vi "REACTOR_MODO AUTOM.vi"(7 "Secuencia":string[](array[string]), 8 "error in (no error)":errorcluster, 9 "ALICATS":T4=[["3", "NO", "M0000013", "Air", "10", "ln/mn", "0", "0"], ["4", "NO", "M0000014", "Air", "10", "ln/mn", "0", "0"], ["5", "NO", "M0000015", "Air", "10", "ln/mn", "0", "0"], ["6", "NO", "M0000016", "Air", "10", "ln/mn", "0", "0"], ["7", "NO", "M0000017", "Air", "10", "ln/mn", "0", "0"], ["8", "NO", "M0000018", "Air", "10", "ln/mn", "0", "0"]], 10 "Eurotherm":T1, 11 "Comms":T5={"Alicats"="ASRL6::INSTR", "Alic"=FALSE, "eValve"="ASRL6::INSTR", "eval"=FALSE, "Eurotherm"="ASRL6::INSTR", "euro"=FALSE, "Cell GAS"="ASRL6::INSTR", "cgas"=FALSE, "Cell H2S"="ASRL6::INSTR", "ch2s"=FALSE}) -> (0 "error out":errorcluster)   [LabVIEW 2017]
uses:
  REACTOR_DATOS.ctl
  REACTOR_COMUNICACIONES.ctl
  SERIAL ALICATS/__s_TablaAlicats.ctl
  EUROTHERM/TEG P116x2.ctl
  EUROTHERM/2xP116.ctl
  SERIAL ALICATS/__Alicat SD_ReadingCluster.ctl
  DISPLAY/Data Type.ctl
  DISPLAY/Display_Command Control.ctl
  REACTOR_MODO AUTOM.ctl
  FILE/File_Module Control.ctl
  TIMING/Timing_Module Control.ctl
  SERIAL RASP_PICO VALVE/kissia_rasPico Module.ctl
  EUROTHERM/Eurotherm_New_Module.ctl
  REACTOR_GLOBALES.vi
panel:
  out "ERRORES_T 2":i32=5 caption="Elapsed Time (s)"
  out "P116x2":T1
  out "ERRORES_T":i32=5 caption="Elapsed Time (s)"
  out "tPlato(s)":dbl=1.0
  out "ParsedReadingArray":T3[](array[typedef]) {"Total" format="%.2f"; "SetPoint" format="%.2f"; "Mass" format="%.2f"; "Volumetric" format="%.2f"; "Temperature" format="%.2f"; "Pressure" format="%.2f"}
  out "T.Wait Stability":bool
  out "Mide Alicats":bool=TRUE
  out "Mide Temps":bool=TRUE
  out "Muestreo(s)":dbl=1.0
  out "TIEMPO (m)":dbl
  out "VALVULA":bool
  out "Timestring":string
  out "Max_t(s)":dbl format="%.1f"
  out "Delta t(s)":dbl format="%.1f"
  out "Delta T(C)":dbl format="%.1f"
  out "TStable":bool
  out "Datos":T6 {"a FSET4" format="%.2g"; "a FSET3" format="%.2g"; "a FSET2" format="%.2g"; "a FSET1" format="%.2g"; "a FLUJO4" format="%.2g"; "a FLUJO2" format="%.2g"; "a FLUJO1" format="%.2g"; "a FLUJO3" format="%.2g"; "eVAL_5" format="%.2g"; "TEMP_TH" format="%.2g"; "SET_TH" format="%.2g"; "TEMP_TC" format="%.2g"; "SET_TC" format="%.2g"; "TIEMPO" format="%.2g"}
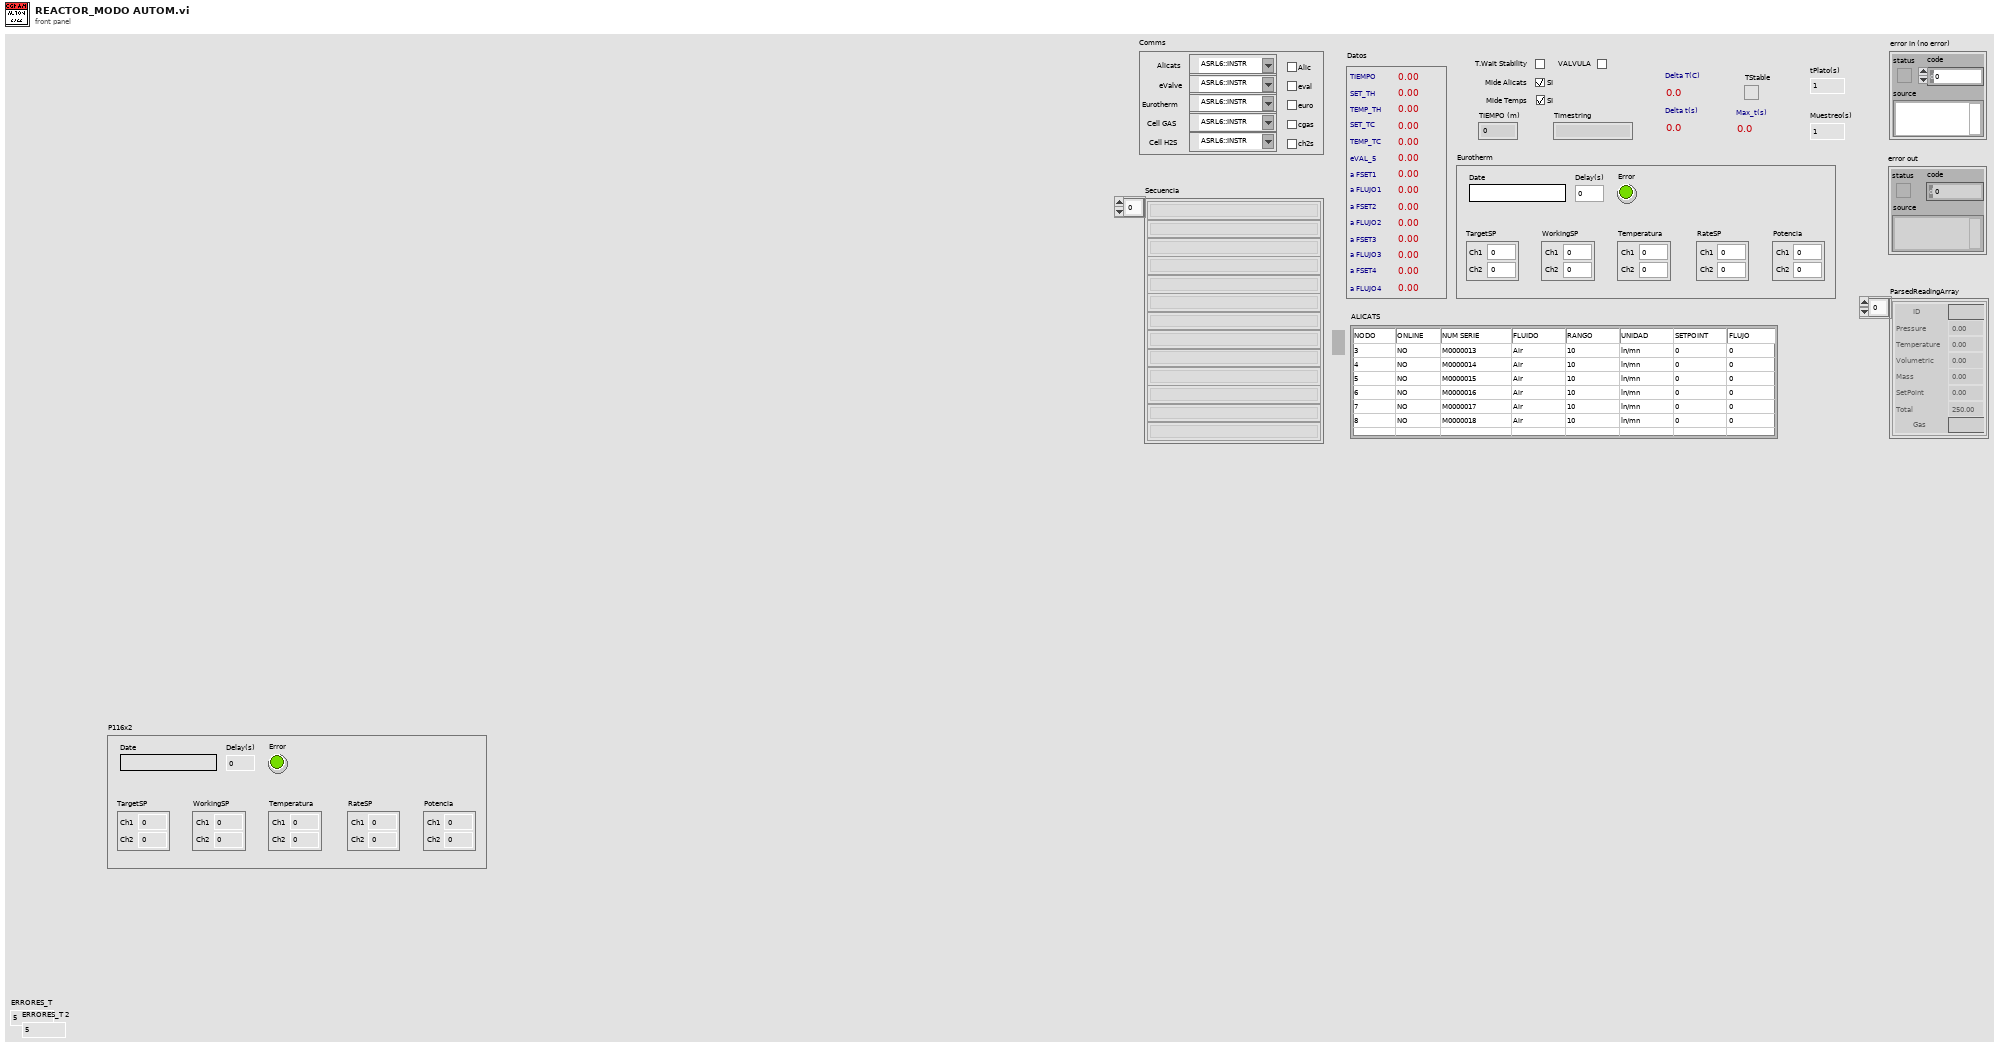
[diagram p1: front panel]
types:
  T1 = typedef "TEG P116x2.ctl" = cluster{"TargetSP":T2, "WorkingSP":T2, "Temperatura":T2, "Error":bool, "Date":string, "Delay(s)":dbl, "RateSP":T2, "Potencia":T2}
  T2 = typedef "2xP116.ctl" = cluster{"Ch1":dbl, "Ch2":dbl}
  T3 = typedef "__Alicat SD_ReadingCluster.ctl" = cluster{"ID":string, "Pressure":sgl, "Temperature":sgl, "Volumetric":sgl, "Mass":sgl, "SetPoint":sgl, "Gas":string, "Total":sgl}
  T4 = typedef "__s_TablaAlicats.ctl" = string[][]
  T5 = typedef "REACTOR_COMUNICACIONES.ctl" = cluster{"Alicats":refnum<visa-resource-name>, "Alic":bool, "eValve":refnum<visa-resource-name>, "eval":bool, "Eurotherm":refnum<visa-resource-name>, "euro":bool, "Cell GAS":refnum<visa-resource-name>, "cgas":bool, "Cell H2S":refnum<visa-resource-name>, "ch2s":bool}
  T6 = typedef "REACTOR_DATOS.ctl" = cluster{"TIEMPO":dbl, "SET_TH":dbl, "TEMP_TH":dbl, "SET_TC":dbl, "TEMP_TC":dbl, "eVAL_5":dbl, "a FSET1":dbl, "a FLUJO1":dbl, "a FSET2":dbl, "a FLUJO2":dbl, "a FSET3":dbl, "a FLUJO3":dbl, "a FSET4":dbl, "a FLUJO4":dbl}
  T7 = typedef "Data Type.ctl" = enum16{"Init FP", "En/Dis FP Ctls", "Update FP", "Upd Status", "Upd Seq"}
  T8 = typedef "Display_Command Control.ctl" = enum16{"Initialize", "Generate Event", "Shutdown"}
  T9 = typedef "REACTOR_MODO AUTOM.ctl" = enum16{"INICIALIZAR", "TEST COMANDO", "PARAMETROS MEDIDA", "CAMBIO ALICATS", "CAMBIO VALVULA", "CAMBIO TEMPERATURAS", "cTEMPERATURA ESTABLE?", "cLEER TIEMPO", "cLEER TEMPERATURAS", "cLEER ALICATS", "cGUARDAR DATOS", "cWAIT NEXT", "CAMBIO TIEMPOS", "tAGOTADO TIEMPO?", "tLEER TIEMPO", "tLEER TEMPERATURAS", "tLEER ALICATS", "tGUARDAR DATOS", "tWAIT NEXT", "FINALIZAR"}
  T10 = typedef "File_Module Control.ctl" = enum16{"Initialize", "Save Head", "Save Data", "Shutdown"}
  T11 = typedef "kissia_rasPico Module.ctl" = enum16{"Initialize", "Read Data", "Write Data", "Enable", "Disable", "Shutdown"}
  T12 = typedef "Timing_Module Control.ctl" = enum16{"Initialize Time", "Check Time"}
  T13 = typedef "Eurotherm_New_Module.ctl" = enum16{"Initialize", "Write SP", "Read SP+PV", "Write Rate", "Set P", "Set I", "Set D", "Shutdown"}
  T14 = typedef "__s_SPali4.ctl" = cluster{"Ch1":dbl, "Ch2":dbl, "Ch3":dbl, "Ch4":dbl, "Ch5":dbl, "Ch6":dbl}
  T15 = enum16{"Add 1", "Add 2", "Add 10", "Add 11", "Add 12", "Add 13"}[]
  T16 = cluster{"processVal":dbl, "targetSP":dbl, "workingSP":dbl, "workingOut":dbl}
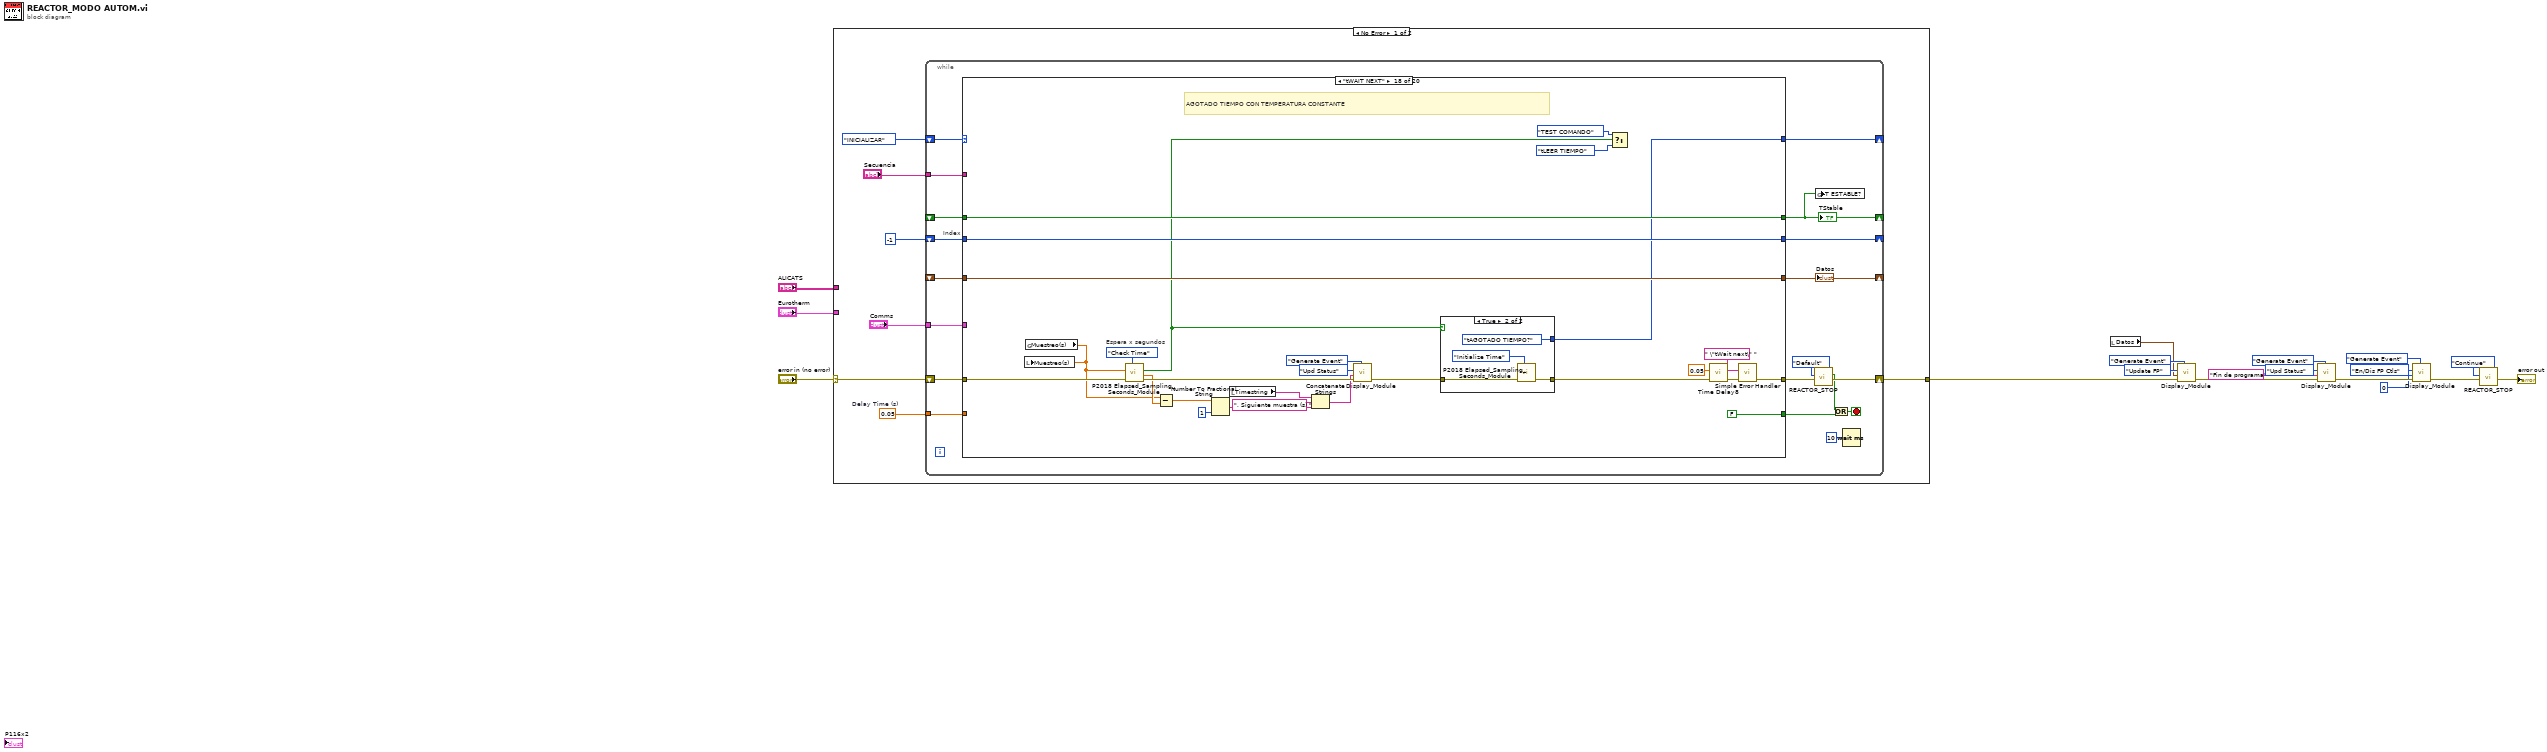
[diagram p0: block diagram]
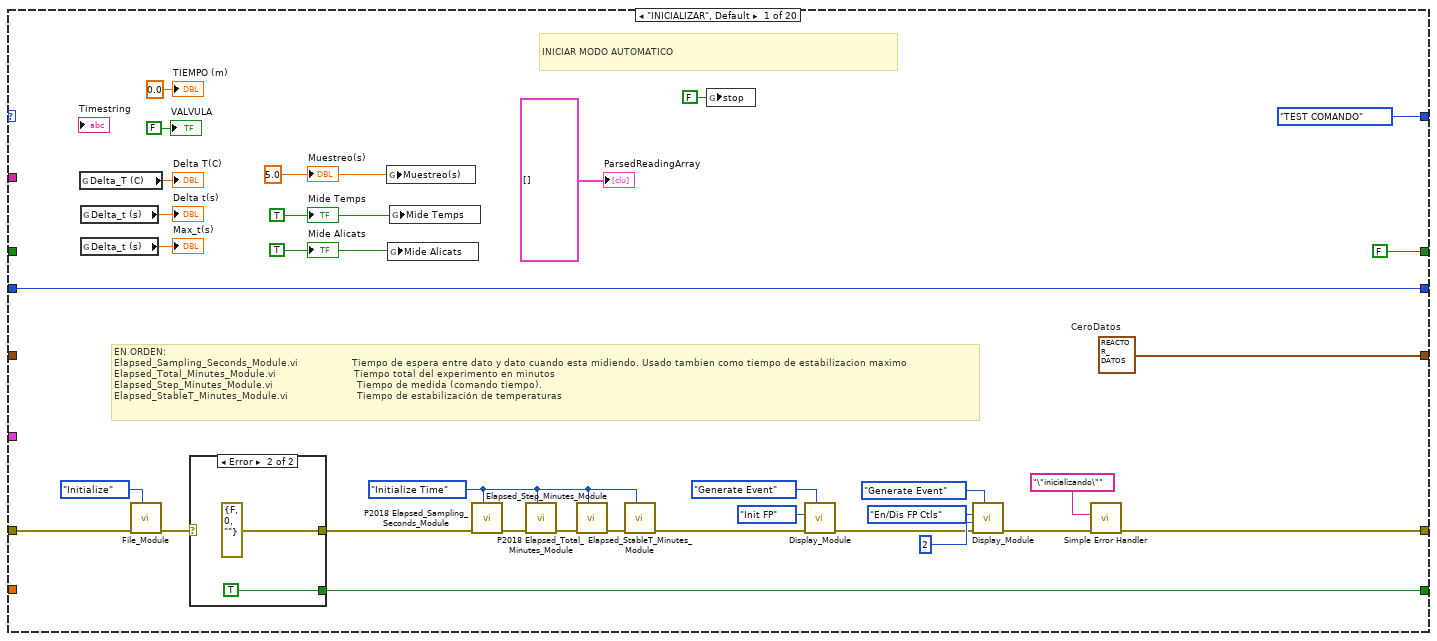
[diagram p2: hidden frame]
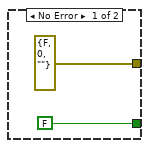
[diagram p3: hidden frame]
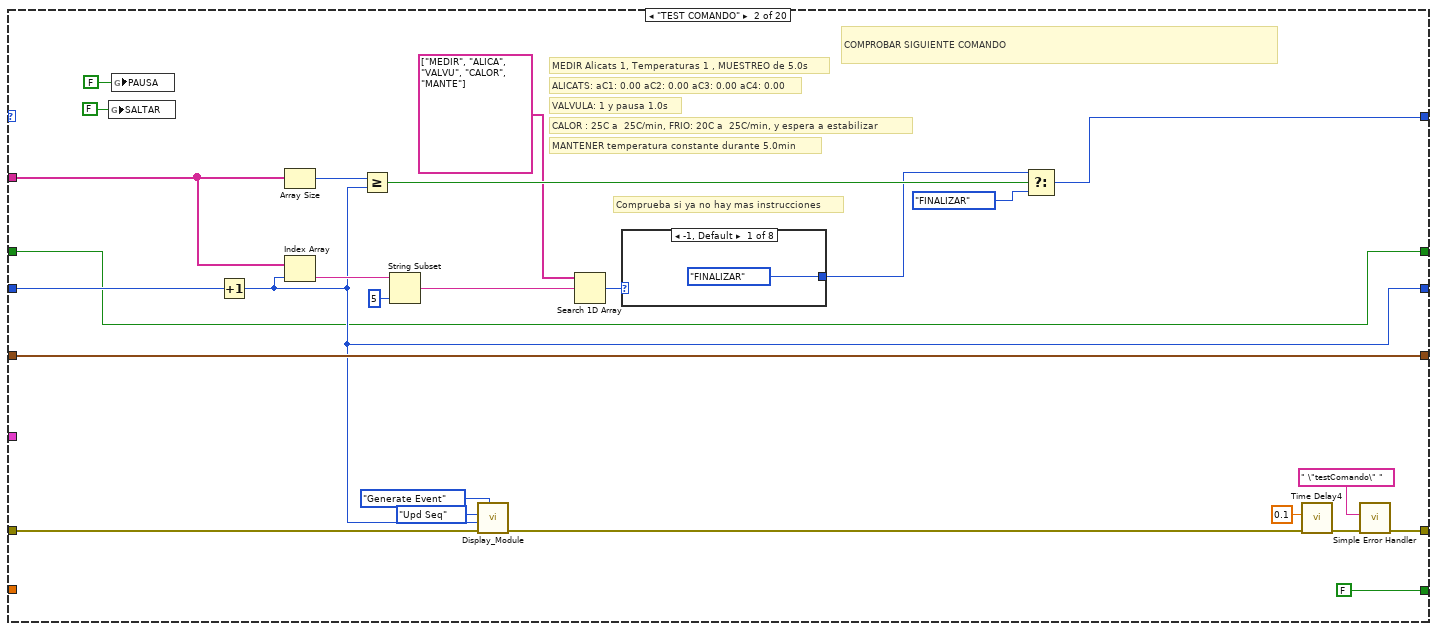
[diagram p4: hidden frame]
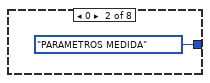
[diagram p5: hidden frame]
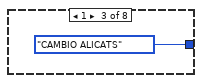
[diagram p6: hidden frame]
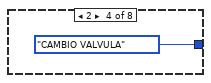
[diagram p7: hidden frame]
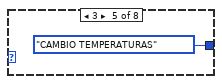
[diagram p8: hidden frame]
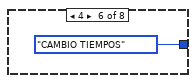
[diagram p9: hidden frame]
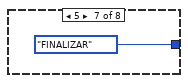
[diagram p10: hidden frame]
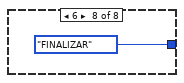
[diagram p11: hidden frame]
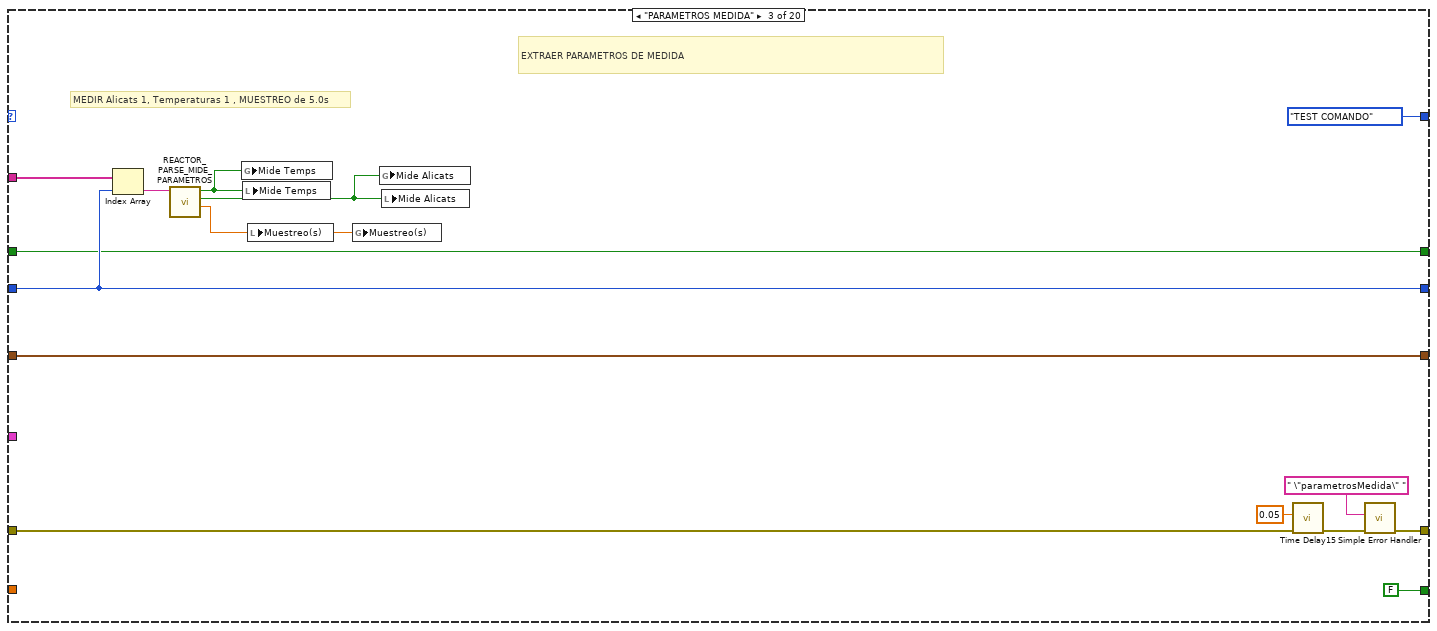
[diagram p12: hidden frame]
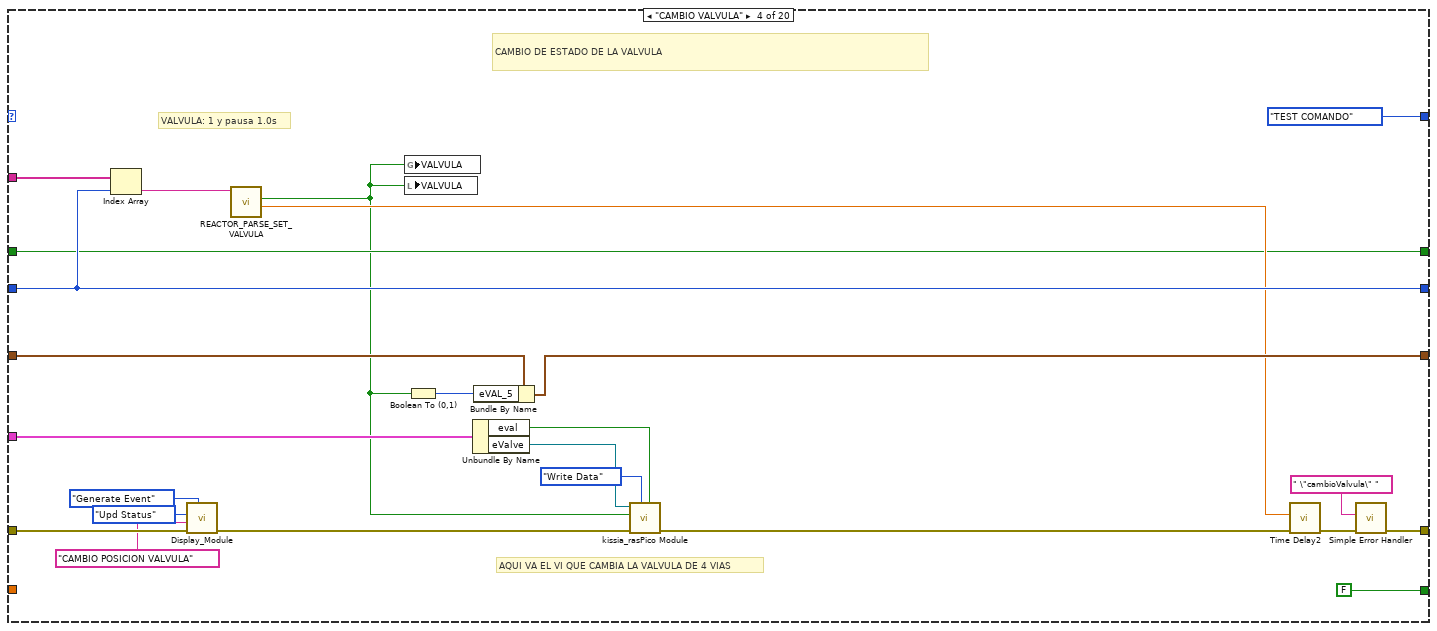
[diagram p13: hidden frame]
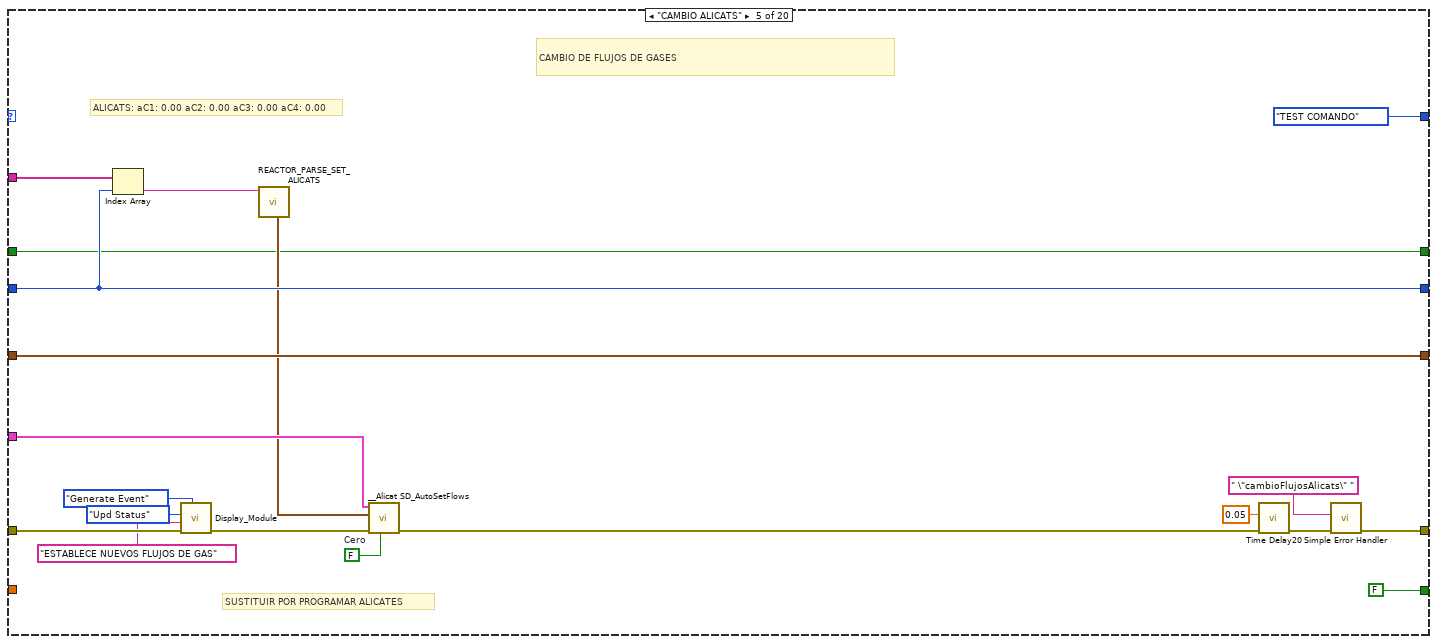
[diagram p14: hidden frame]
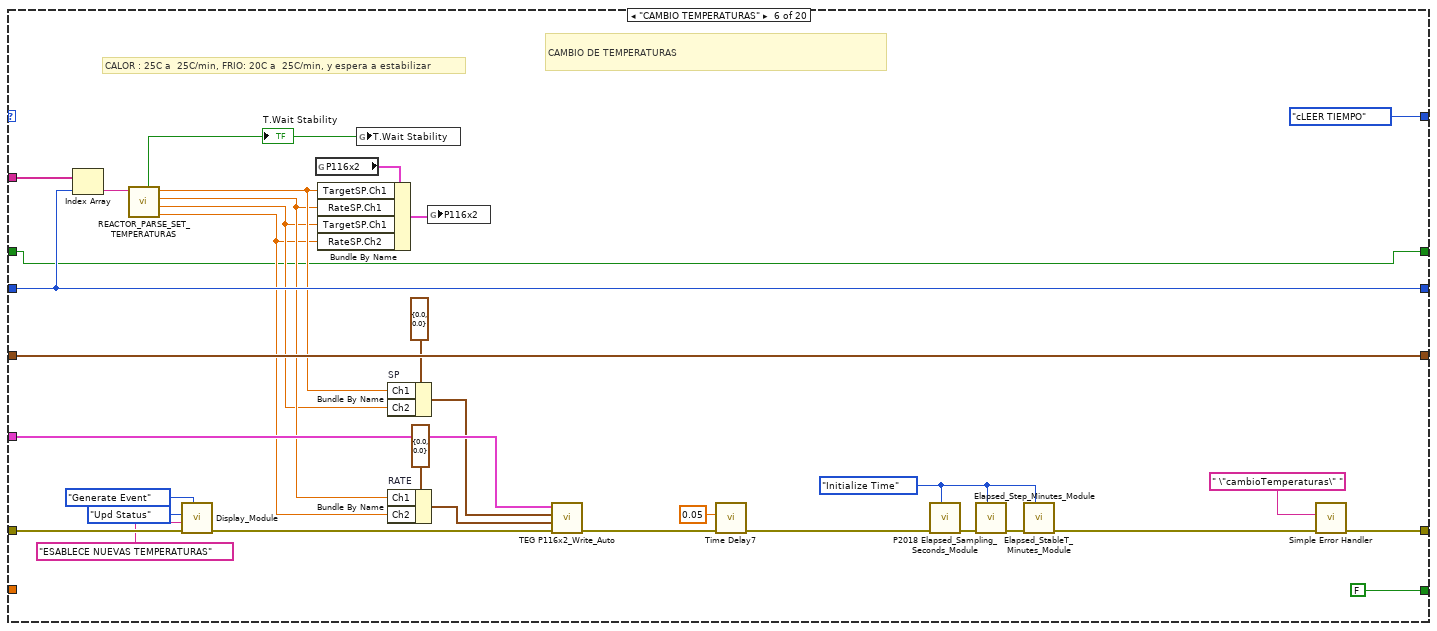
[diagram p15: hidden frame]
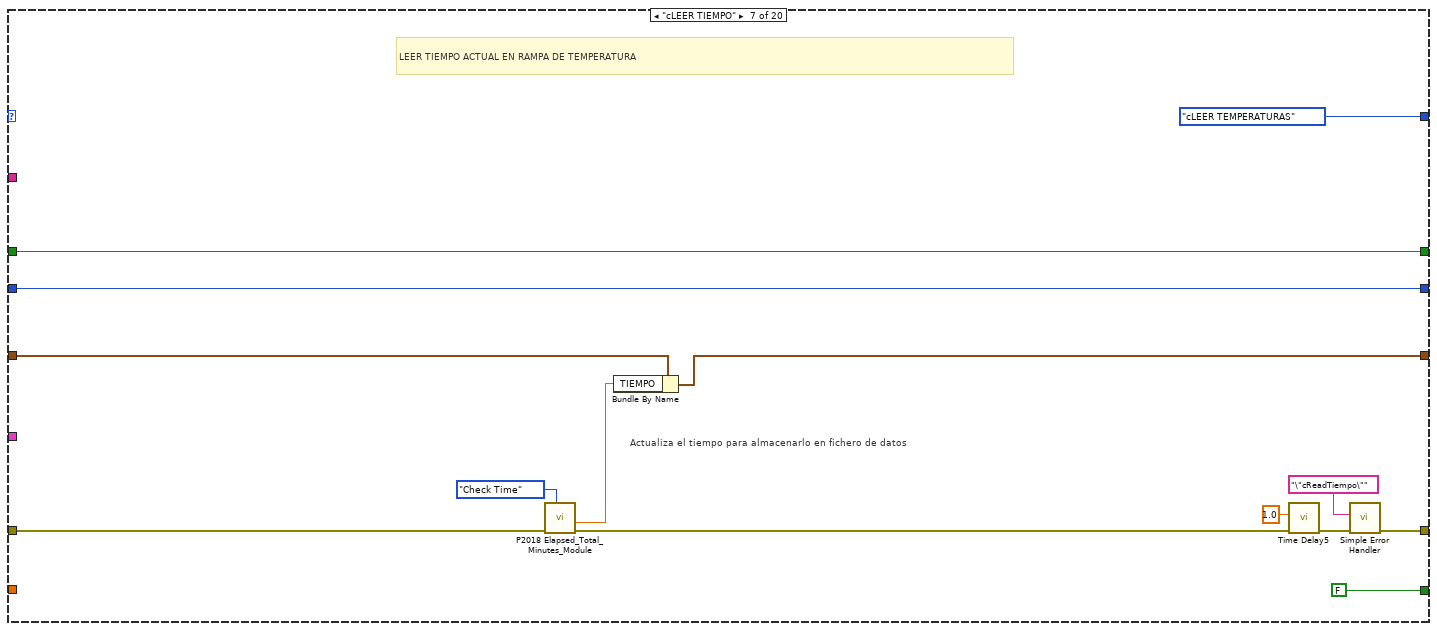
[diagram p16: hidden frame]
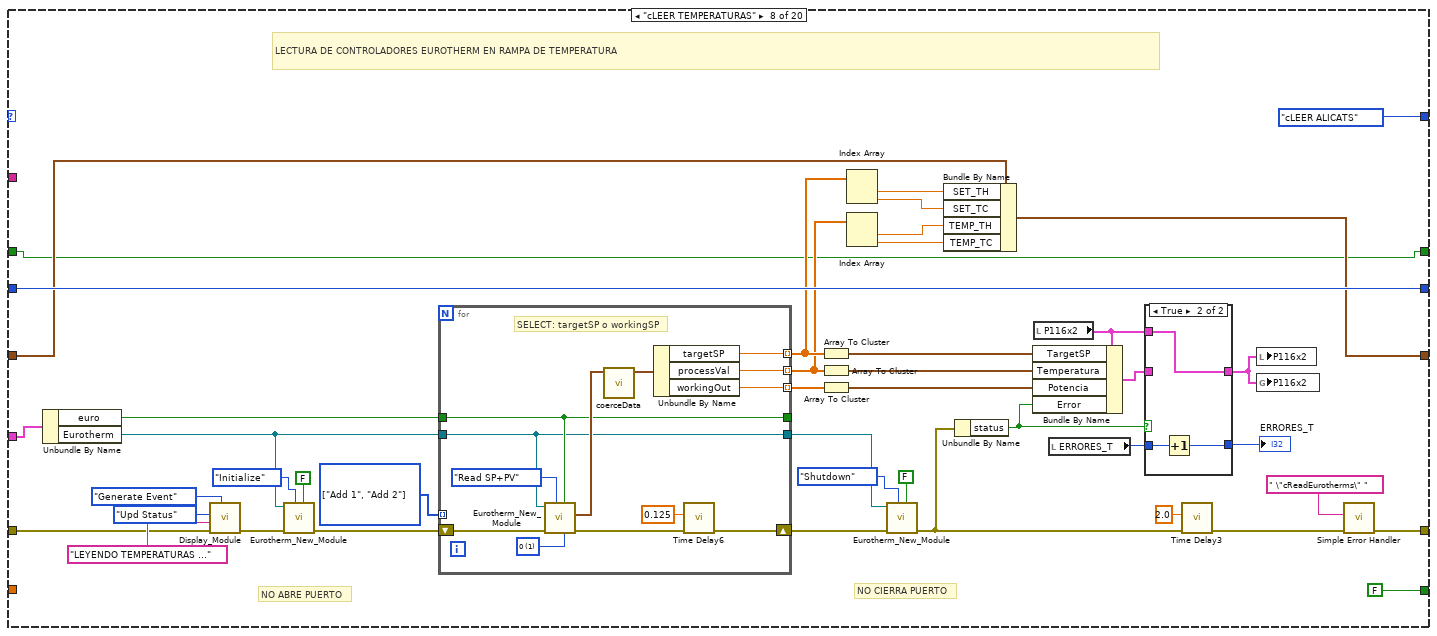
[diagram p17: hidden frame]
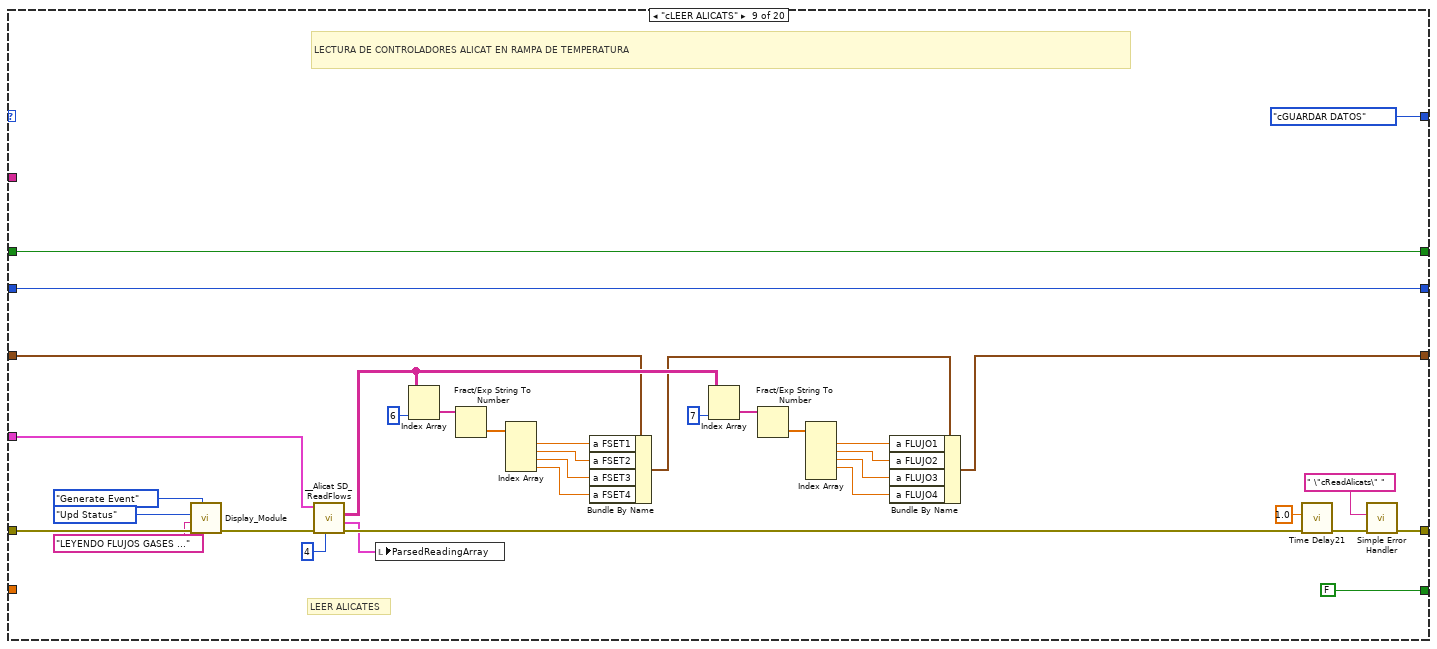
[diagram p19: hidden frame]
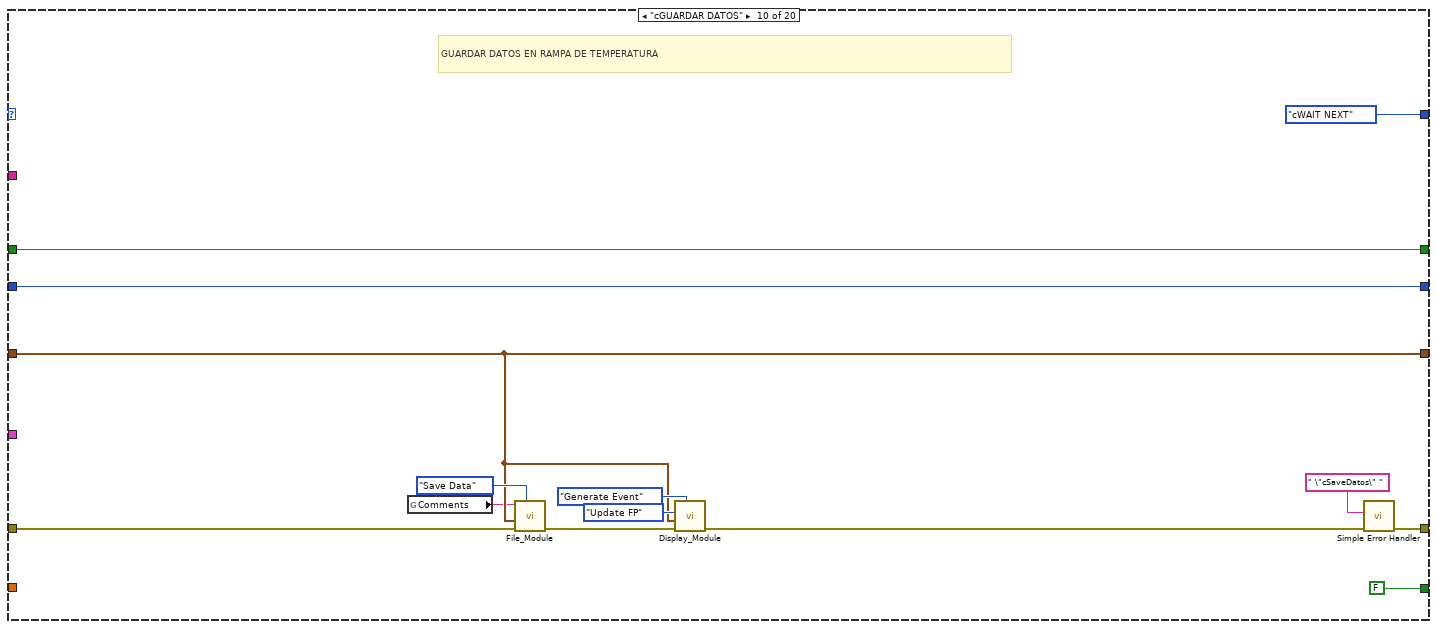
[diagram p20: hidden frame]
diagram:
  n1 = case shown="No Error" "error in (no error)" {
    selector: "error in (no error)" -> [w25 w636]
    tunnel: [w24 w636] -> w1
    tunnel: "Eurotherm" -> [_ _]
    tunnel: "ALICATS" -> [_ _]
    frame No Error {
      w19 = 0.05  # Delay Time (s)
      n2 = while {
        shift-right: [w39] -> _
        shift-left: REACTOR_MODO_AUTOM."INICIALIZAR" ("Command") -> [w40]
        shift-right: [w27] -> w24
        shift-left: w25 -> [w41]
        shift-right: [w34] -> _
        shift-left: _ -> [w38]
        tunnel: "Secuencia" -> [w37]
        shift-right: [w35] -> _
        shift-left: -1 ("milliseconds to wait") -> [w36]
        tunnel: "Comms" -> [w33]
        shift-right: [w31] -> _
        shift-left: _ -> [w32]
        tunnel: w19 -> [w30]
        stop <- w43 stop-if-true
        # "Index"
        n3 = case shown="\"tWAIT NEXT\"" w40 {
          tunnel: [w65 FALSE FALSE FALSE FALSE FALSE FALSE FALSE FALSE FALSE FALSE FALSE FALSE FALSE FALSE FALSE FALSE FALSE FALSE TRUE] -> w42
          tunnel: w41 -> [w76 w91 w121 w152 w172 w205 w217 w228 w315 w331 w352 w367 w422 w439 w450 w537 w555 w577 w613 w630]
          tunnel: [w60 w85 w126 w143 w166 w195 w213 w223 w312 w320 w333 w371 w418 w435 w445 w534 w545 w565 w598 w621] -> w28
          tunnel: [REACTOR_MODO_AUTOM."TEST COMANDO" ("Command") w102 REACTOR_MODO_AUTOM."TEST COMANDO" ("Command") REACTOR_MODO_AUTOM."TEST COMANDO" ("Command") REACTOR_MODO_AUTOM."TEST COMANDO" ("Command") REACTOR_MODO_AUTOM."cLEER TIEMPO" ("Command") REACTOR_MODO_AUTOM."cLEER TEMPERATURAS" ("Command") REACTOR_MODO_AUTOM."cLEER ALICATS" ("Command") REACTOR_MODO_AUTOM."cGUARDAR DATOS" ("Command") REACTOR_MODO_AUTOM."cWAIT NEXT" ("Command") w355 w398 REACTOR_MODO_AUTOM."tLEER TIEMPO" ("Command") REACTOR_MODO_AUTOM."tLEER TEMPERATURAS" ("Command") REACTOR_MODO_AUTOM."tLEER ALICATS" ("Command") REACTOR_MODO_AUTOM."tGUARDAR DATOS" ("Command") REACTOR_MODO_AUTOM."tWAIT NEXT" ("Command") w557 w589 REACTOR_MODO_AUTOM."FINALIZAR" ("Command")] -> w39
          tunnel: [w75 w106 w120 w146 w162 w201 w218 w226 w285 w324 w354 w373 w425 w440 w448 w507 w548 w579 w615 w634] -> w34
          tunnel: w38 -> [_ w106 w120 w147 w162 w201 w221 w227 w287 w324 w354 w373 w425 w443 w449 w509 w548 w579 w615 w634]
          tunnel: w37 -> [_ w105 w130 w154 w174 w207 _ _ _ _ _ _ w427 _ _ _ _ _ _ _]
          tunnel: w36 -> [w71 w95 w129 w150 w170 w203 w219 w263 w316 w328 w343 w399 w426 w441 w485 w538 w552 w570 w607 w633]
          tunnel: [w71 w93 w129 w150 w170 w203 w219 w263 w316 w328 w343 w399 w426 w441 w485 w538 w552 w570 w607 w633] -> w35
          tunnel: w33 -> [_ _ _ w134 w158 w186 _ w224 w306 _ _ _ _ _ w446 w528 _ _ _ _]
          tunnel: w32 -> [_ w82 w116 w133 w155 w175 w215 w222 w314 w323 w336 _ w420 w437 w444 w536 w547 w568 w600 w624]
          tunnel: [FALSE ("TStable?") w82 w116 w133 w155 w175 w215 w222 w314 w323 w336 w376 w420 w437 w444 w536 w547 w568 w600 w624] -> w31
          tunnel: w30 -> [_ _ _ _ _ _ _ _ _ _ _ _ _ _ _ _ _ _ _ _]
          frame "INICIALIZAR", Default {
            w49 = TRUE ("Mide Temps")
            w48 = TRUE ("Mide Alicats")
            w47 = 5.0 ("Sampling(s)")
            w56 = Timing_Module_Control."Initialize Time" ("Command")
            w75 = T6 {"TIEMPO"=0.0, "SET_TH"=0.0, "TEMP_TH"=0.0, "SET_TC"=0.0, "TEMP_TC"=0.0, "eVAL_5"=0.0, "a FSET1"=0.0, "a FLUJO1"=0.0, "a FSET2"=0.0, "a FLUJO2"=0.0, "a FSET3"=0.0, "a FLUJO3"=0.0, "a FSET4"=0.0, "a FLUJO4"=0.0}  # CeroDatos
            # "INICIAR MODO AUTOMATICO"
            # "EN ORDEN:\nElapsed_Sampling_Seconds_Module.vi                  Tiempo de espera entre dato y dato cuando esta midiendo. Usado tambien como tiempo de estabilizacion maximo \nElapsed_Total_Minutes_Module.vi                          Tiempo total del experimento en minutos\nElapsed_Step_Minutes_Module.vi                            Tiempo de medida (comando tiempo). \nElapsed_StableT_Minutes_Module.vi                       Tiempo de estabilización de temperaturas"
            n4 = global read "REACTOR_GLOBALES.vi" "Delta_T (C)"() -> (→"Delta T(C)":dbl)
            n5 = global read "REACTOR_GLOBALES.vi" "Delta_t (s)"() -> (→"Delta t(s)":dbl)
            n6 = global read "REACTOR_GLOBALES.vi" "Delta_t (s)"() -> (→"Max_t(s)":dbl)
            n7 = call "File_Module.vi"("Command"=File_Module_Control."Initialize", "error in (no error)"=w76) -> ("error out"=w67:errorcluster)  [unwired: 8 in, 1 out]
            n8 = case shown="Error" w67 {
              tunnel: [errorcluster {"status"=FALSE, "code"=0, "source"=""} ("error out") errorcluster {"status"=FALSE, "code"=0, "source"=""} ("error out")] -> w66
              tunnel: [FALSE TRUE] -> w65
              frame No Error {
              }
              frame Error {
              }
            }
            n9 = global write "REACTOR_GLOBALES.vi" "Muestreo(s)"(w47) -> ()
            n10 = global write "REACTOR_GLOBALES.vi" "Mide Alicats"(w48) -> ()
            n11 = global write "REACTOR_GLOBALES.vi" "Mide Temps"(w49) -> ()
            n12 = call "P2018 Elapsed_Sampling_Seconds_Module.vi"("Command"=w56, "error in (no error)"=w66) -> ("error out"=w64:errorcluster)  [unwired: 7 in, 2 out]
            n13 = call "P2018 Elapsed_Total_Minutes_Module.vi"("Command"=w56, "error in (no error)"=w64) -> ("error out"=w63:errorcluster)  [unwired: 7 in, 2 out]
            n14 = call "Elapsed_Step_Minutes_Module.vi"("Command"=w56, "error in (no error)"=w63) -> ("error out"=w58:errorcluster)  [unwired: 7 in, 2 out]
            n15 = call "Elapsed_StableT_Minutes_Module.vi"("Command"=w56, "error in (no error)"=w58) -> ("error out"=w57:errorcluster)  [unwired: 7 in, 2 out]
            n16 = global write "REACTOR_GLOBALES.vi" "stop"(FALSE ("stop")) -> ()
            n17 = call "Display_Module.vi"("Command"=Display_Command_Control."Generate Event", "error in (no error)"=w57, "Data Type"=Data_Type."Init FP") -> ("error out"=w68:errorcluster)  [unwired: 8 in]
            n18 = call "Display_Module.vi"("Command"=Display_Command_Control."Generate Event", "error in (no error)"=w68, "Data"=2, "Data Type"=Data_Type."En/Dis FP Ctls") -> ("error out"=w61:errorcluster)  [unwired: 7 in]
            n19 = call <vilib>:"Simple Error Handler.vi"("error source (\" \")"="\"inicializando\"" ("error source (\" \")"), "error in (no error)"=w61) -> ("error out"=w60:errorcluster)  [unwired: 3 in, 4 out]
            "TIEMPO (m)" <- 0.0 ("TIEMPO (m)")
            "VALVULA" <- FALSE ("VALVULA")
            "Muestreo(s)" <- w47
            "Mide Alicats" <- w48
            "Mide Temps" <- w49
            "ParsedReadingArray" <- T3[] [] ("ParsedReadingArray")
          }
          frame "TEST COMANDO" {
            # "COMPROBAR SIGUIENTE COMANDO"
            # "MEDIR Alicats 1, Temperaturas 1 , MUESTREO de 5.0s"
            # "VALVULA: 1 y pausa 1.0s"
            # "CALOR : 25C a  25C/min, FRIO: 20C a  25C/min, y espera a estabilizar"
            # "MANTENER temperatura constante durante 5.0min"
            # "ALICATS: aC1: 0.00 aC2: 0.00 aC3: 0.00 aC4: 0.00"
            # "Comprueba si ya no hay mas instrucciones"
            n20 = global write "REACTOR_GLOBALES.vi" "SALTAR"(FALSE ("Saltar")) -> ()
            n21 = global write "REACTOR_GLOBALES.vi" "PAUSA"(FALSE ("Saltar")) -> ()
            n22 = Increment(x=w95) -> (x+1=w93:i32)
            n23 = Array Size(array=w105) -> (size(s)=w104:i32)
            n24 = Index Array(array=w105, index=w93) -> (element=w100:string)
            n25 = Greater Or Equal?(x=w104, y=w93) -> (x >= y?=w103:bool)
            n26 = String Subset(string=w100, length (rest)=5 ("length (rest)")) -> (substring=w98:string)  [unwired: 1 in]
            n27 = call "Display_Module.vi"("Command"=Display_Command_Control."Generate Event", "error in (no error)"=w91, "Data"=w93, "Data Type"=Data_Type."Upd Seq") -> ("error out"=w88:errorcluster)  [unwired: 7 in]
            n28 = Search 1D Array(1D array=string[] ["MEDIR", "ALICA", "VALVU", "CALOR", "MANTE"], element=w98) -> (index of element=w97:i32)  [unwired: 1 in]
            n29 = case shown="-1, Default" w97 {
              tunnel: [REACTOR_MODO_AUTOM."FINALIZAR" ("Command") REACTOR_MODO_AUTOM."PARAMETROS MEDIDA" ("Command") REACTOR_MODO_AUTOM."CAMBIO ALICATS" ("Command") REACTOR_MODO_AUTOM."CAMBIO VALVULA" ("Command") REACTOR_MODO_AUTOM."CAMBIO TEMPERATURAS" ("Command") REACTOR_MODO_AUTOM."CAMBIO TIEMPOS" ("Command") REACTOR_MODO_AUTOM."FINALIZAR" ("Command") REACTOR_MODO_AUTOM."FINALIZAR" ("Command")] -> w96
              frame -1, Default {
              }
              frame 0 {
              }
              frame 1 {
              }
              frame 2 {
              }
              frame 3 {
              }
              frame 4 {
              }
              frame 5 {
              }
              frame 6 {
              }
            }
            n30 = Select(t=w96, s=w103, f=REACTOR_MODO_AUTOM."FINALIZAR" ("Command")) -> (s? t:f=w102:T9)
            n31 = call "Time Delay4"("error in (no error)"=w88, "Delay Time (s)"=0.1) -> ("error out"=w86:errorcluster)  [unwired: 9 in]
            n32 = call <vilib>:"Simple Error Handler.vi"("error source (\" \")"=" \"testComando\" " ("error source (\" \")"), "error in (no error)"=w86) -> ("error out"=w85:errorcluster)  [unwired: 3 in, 4 out]
          }
          frame "PARAMETROS MEDIDA" {
            # "EXTRAER PARAMETROS DE MEDIDA"
            # "MEDIR Alicats 1, Temperaturas 1 , MUESTREO de 5.0s"
            n33 = Index Array(array=w130, index=w129) -> (element=w123:string)
            n34 = call "REACTOR_PARSE_MIDE_PARAMETROS.vi"("String"=w123) -> ("Pausa (s)"=w117:dbl, "Mide Alicats"=w118:bool, "Mide Eurotherm"=w119:bool)  [unwired: 8 in]
            n35 = global write "REACTOR_GLOBALES.vi" "Mide Temps"(w119) -> ()
            n36 = local write "Mide Temps"(w119) -> ()
            n37 = local write "Muestreo(s)"(w117) -> ()
            n38 = global write "REACTOR_GLOBALES.vi" "Muestreo(s)"(w117) -> ()
            n39 = global write "REACTOR_GLOBALES.vi" "Mide Alicats"(w118) -> ()
            n40 = local write "Mide Alicats"(w118) -> ()
            n41 = call "Time Delay15"("error in (no error)"=w121, "Delay Time (s)"=0.05) -> ("error out"=w124:errorcluster)  [unwired: 9 in]
            n42 = call <vilib>:"Simple Error Handler.vi"("error source (\" \")"=" \"parametrosMedida\" " ("error source (\" \")"), "error in (no error)"=w124) -> ("error out"=w126:errorcluster)  [unwired: 3 in, 4 out]
          }
          frame "CAMBIO VALVULA" {
            # "CAMBIO DE ESTADO DE LA VALVULA"
            # "VALVULA: 1 y pausa 1.0s"
            # "AQUI VA EL VI QUE CAMBIA LA VALVULA DE 4 VIAS"
            n43 = Index Array(array=w154, index=w150) -> (element=w142:string)
            n44 = call "Display_Module.vi"("Command"=Display_Command_Control."Generate Event", "error in (no error)"=w152, "Data"="CAMBIO POSICION VALVULA" ("element"), "Data Type"=Data_Type."Upd Status") -> ("error out"=w136:errorcluster)  [unwired: 7 in]
            n45 = call "REACTOR_PARSE_SET_VALVULA.vi"("String"=w142) -> ("Pausa (s)"=w141:dbl, "VALVULA 1"=w132:bool)  [unwired: 9 in]
            n46 = global write "REACTOR_GLOBALES.vi" "VALVULA"(w132) -> ()
            n47 = local write "VALVULA"(w132) -> ()
            n48 = Boolean To (0,1)(Boolean=w132) -> (0, 1=w131:i16)
            n49 = Unbundle By Name(w134) -> ("eval"=w139:bool, "eValve"=w137:refnum<visa-resource-name>)
            n50 = Bundle By Name(cluster=w147, "eVAL_5"=w131) -> (w146:T6)
            n51 = call "kissia_rasPico Module.vi"("Enable"=w139, "Command"=kissia_rasPico_Module."Write Data", "error in (no error)"=w136, "VALVE"=w132, "VISA resource name"=w137) -> ("error out"=w135:errorcluster)  [unwired: 3 in, 3 out]
            n52 = call "Time Delay2"("error in (no error)"=w135, "Delay Time (s)"=w141) -> ("error out"=w144:errorcluster)  [unwired: 9 in]
            n53 = call <vilib>:"Simple Error Handler.vi"("error source (\" \")"=" \"cambioValvula\" " ("error source (\" \")"), "error in (no error)"=w144) -> ("error out"=w143:errorcluster)  [unwired: 3 in, 4 out]
          }
          frame "CAMBIO ALICATS" {
            w160 = FALSE  # Cero
            # "CAMBIO DE FLUJOS DE GASES"
            # "ALICATS: aC1: 0.00 aC2: 0.00 aC3: 0.00 aC4: 0.00"
            # "SUSTITUIR POR PROGRAMAR ALICATES"
            n54 = Index Array(array=w174, index=w170) -> (element=w163:string)
            n55 = call "Display_Module.vi"("Command"=Display_Command_Control."Generate Event", "error in (no error)"=w172, "Data"="ESTABLECE NUEVOS FLUJOS DE GAS" ("element"), "Data Type"=Data_Type."Upd Status") -> ("error out"=w159:errorcluster)  [unwired: 7 in]
            n56 = call "REACTOR_PARSE_SET_ALICATS.vi"("String"=w163) -> ("ALICATS_SP"=w157:T14)  [unwired: 6 in, 4 out]
            n57 = call "__Alicat SD_AutoSetFlows.vi"("Cero"=w160, "error in (no error)"=w159, "ALICATS_SP"=w157, "COMMS"=w158) -> ("error out"=w161:errorcluster)  [unwired: 7 in]
            n58 = call "Time Delay20"("error in (no error)"=w161, "Delay Time (s)"=0.05) -> ("error out"=w164:errorcluster)  [unwired: 9 in]
            n59 = call <vilib>:"Simple Error Handler.vi"("error source (\" \")"=" \"cambioFlujosAlicats\" " ("error source (\" \")"), "error in (no error)"=w164) -> ("error out"=w166:errorcluster)  [unwired: 3 in, 4 out]
          }
          frame "CAMBIO TEMPERATURAS" {
            w194 = Timing_Module_Control."Initialize Time" ("Command")
            # "CAMBIO DE TEMPERATURAS"
            # "CALOR : 25C a  25C/min, FRIO: 20C a  25C/min, y espera a estabilizar"
            n60 = Index Array(array=w207, index=w203) -> (element=w190:string)
            n61 = call "REACTOR_PARSE_SET_TEMPERATURAS.vi"("String"=w190) -> ("RAMPA_F (C/MIN)"=w177:dbl, "FRIO (C)"=w178:dbl, "RAMPA_C (C/MIN)"=w179:dbl, "CALOR (C)"=w180:dbl, "T.Wait Stability"=w187:bool)  [unwired: 6 in]
            "T.Wait Stability" <- w187
            n62 = call "Display_Module.vi"("Command"=Display_Command_Control."Generate Event", "error in (no error)"=w205, "Data"="ESABLECE NUEVAS TEMPERATURAS" ("element"), "Data Type"=Data_Type."Upd Status") -> ("error out"=w185:errorcluster)  [unwired: 7 in]
            n63 = global read "REACTOR_GLOBALES.vi" "P116x2"() -> (w188:T1)
            n64 = Bundle By Name(cluster=w188, "TargetSP.Ch1"=w180, "RateSP.Ch1"=w179, "TargetSP.Ch1"=w178, "RateSP.Ch2"=w177) -> (w189:T1)
            n65 = global write "REACTOR_GLOBALES.vi" "T.Wait Stability"(w187) -> ()
            n66 = Bundle By Name "SP"(cluster=T2 {"Ch1"=0.0, "Ch2"=0.0} ("NuevoSP"), "Ch1"=w180, "Ch2"=w178) -> (w181:T2)
            n67 = Bundle By Name "RATE"(cluster=T2 {"Ch1"=0.0, "Ch2"=0.0} ("NuevoSP"), "Ch1"=w179, "Ch2"=w177) -> (w182:T2)
            n68 = global write "REACTOR_GLOBALES.vi" "P116x2"(w189) -> ()
            n69 = call "TEG P116x2_Write_Auto.vi"("error in (no error)"=w185, "NuevoRT"=w182, "NuevoSP"=w181, "Comunicaciones"=w186) -> ("error out"=w184:errorcluster)  [unwired: 5 in, 2 out]
            n70 = call "Time Delay7"("error in (no error)"=w184, "Delay Time (s)"=0.05) -> ("error out"=w198:errorcluster)  [unwired: 9 in]
            n71 = call "P2018 Elapsed_Sampling_Seconds_Module.vi"("Command"=w194, "error in (no error)"=w198) -> ("error out"=w197:errorcluster)  [unwired: 7 in, 2 out]
            n72 = call "Elapsed_Step_Minutes_Module.vi"("Command"=w194, "error in (no error)"=w197) -> ("error out"=w193:errorcluster)  [unwired: 7 in, 2 out]
            n73 = call "Elapsed_StableT_Minutes_Module.vi"("Command"=w194, "error in (no error)"=w193) -> ("error out"=w192:errorcluster)  [unwired: 7 in, 2 out]
            n74 = call <vilib>:"Simple Error Handler.vi"("error source (\" \")"=" \"cambioTemperaturas\" " ("error source (\" \")"), "error in (no error)"=w192) -> ("error out"=w195:errorcluster)  [unwired: 3 in, 4 out]
          }
          frame "cLEER TIEMPO" {
            # "LEER TIEMPO ACTUAL EN RAMPA DE TEMPERATURA"
            # "Actualiza el tiempo para almacenarlo en fichero de datos"
            n75 = call "P2018 Elapsed_Total_Minutes_Module.vi"("Command"=Timing_Module_Control."Check Time", "error in (no error)"=w217) -> ("error out"=w209:errorcluster, "Elapsed Out"=w212:dbl)  [unwired: 7 in, 1 out]
            n76 = Bundle By Name(cluster=w221, "TIEMPO"=w212) -> (w218:T6)
            n77 = call "Time Delay5"("error in (no error)"=w209, "Delay Time (s)"=1.0) -> ("error out"=w210:errorcluster)  [unwired: 9 in]
            n78 = call <vilib>:"Simple Error Handler.vi"("error source (\" \")"="\"cReadTiempo\"" ("error source (\" \")"), "error in (no error)"=w210) -> ("error out"=w213:errorcluster)  [unwired: 3 in, 4 out]
          }
          frame "cLEER TEMPERATURAS" {
            w233 = T15 [enum."Add 1", enum."Add 2"] items=["Add 1", "Add 2", "Add 10", "Add 11", "Add 12", "Add 13"]
            # "NO CIERRA PUERTO"
            # "NO ABRE PUERTO"
            # "LECTURA DE CONTROLADORES EUROTHERM EN RAMPA DE TEMPERATURA"
            n79 = Unbundle By Name(w224) -> ("euro"=w257:bool, "Eurotherm"=w259:refnum<visa-resource-name>)
            n80 = call "Display_Module.vi"("Command"=Display_Command_Control."Generate Event", "error in (no error)"=w228, "Data"="LEYENDO TEMPERATURAS ...", "Data Type"=Data_Type."Upd Status") -> ("error out"=w246:errorcluster)  [unwired: 7 in]
            n81 = call "Eurotherm_New_Module.vi"("Eurotherm (T:Enable)"=FALSE, "Command"=Eurotherm_New_Module."Initialize", "error in (no error)"=w246, "VISA resource name"=w259) -> ("error out"=w256:errorcluster)  [unwired: 6 in, 1 out]
            n82 = for {
              tunnel: w233 -> [_] mode=indexing
              tunnel: [w282] -> w243 mode=indexing
              tunnel: [w281] -> w242 mode=indexing
              shift-right: [w279] -> w258
              shift-left: w256 -> [w275]
              tunnel: w257 -> [w271]
              tunnel: [w280] -> w255 mode=indexing
              tunnel: [w271] -> _
              tunnel: w259 -> [w270]
              tunnel: [w270] -> w260
              w272 = u16 1 items=["0"=1, "1"=10, "2"=100] ("Decimales")
              # "SELECT: targetSP o workingSP"
              n83 = call "Eurotherm_New_Module.vi"("Decimales"=w272, "Eurotherm (T:Enable)"=w271, "Command"=Eurotherm_New_Module."Read SP+PV", "error in (no error)"=w275, "VISA resource name"=w270) -> ("error out"=w276:errorcluster, "Eurotherm"=w273:T16)  [unwired: 5 in]
              n84 = call "coerceData.vi"("Eurotherm"=w273) -> ("Eurotherm 2"=w277:T16)  [unwired: 10 in]
              n85 = Unbundle By Name(w277) -> ("targetSP"=w282:dbl, "processVal"=w281:dbl, "workingOut"=w280:dbl)
              n86 = call "Time Delay6"("error in (no error)"=w276, "Delay Time (s)"=0.125) -> ("error out"=w279:errorcluster)  [unwired: 9 in]
            }
            n87 = Array To Cluster(array=w243) -> (cluster=w252:cluster{"[0]":dbl, "[1]":dbl})
            n88 = Array To Cluster(array=w242) -> (cluster=w251:cluster{"[0]":dbl, "[1]":dbl})
            n89 = Array To Cluster(array=w255) -> (cluster=w250:cluster{"[0]":dbl, "[1]":dbl})
            n90 = Index Array(array=w243) -> (element #1=w241:dbl, element #2=w240:dbl)  [unwired: 2 in]
            n91 = Index Array(array=w242) -> (element #1=w239:dbl, element #2=w238:dbl)  [unwired: 2 in]
            n92 = call "Eurotherm_New_Module.vi"("Eurotherm (T:Enable)"=FALSE, "Command"=Eurotherm_New_Module."Shutdown", "error in (no error)"=w258, "VISA resource name"=w260) -> ("error out"=w247:errorcluster)  [unwired: 6 in, 1 out]
            n93 = Bundle By Name(cluster=w227, "SET_TH"=w241, "SET_TC"=w240, "TEMP_TH"=w239, "TEMP_TC"=w238) -> (w226:T6)
            n94 = Unbundle By Name(w247) -> ("status"=w254:bool)
            n95 = local read "P116x2"() -> (w244:T1)
            n96 = Bundle By Name(cluster=w244, "TargetSP"=w252, "Temperatura"=w251, "Potencia"=w250, "Error"=w254) -> (w253:T1)
            n97 = local read "ERRORES_T"() -> (w249:i32)
            n98 = case shown="True" w254 {
              tunnel: w253 -> [w266 _]
              tunnel: [w266 w267] -> w245
              tunnel: w244 -> [_ w267]
              tunnel: w249 -> [w265 w269]
              tunnel: [w265 w268] -> w248
              frame False {
              }
              frame True {
                n99 = Increment(x=w269) -> (x+1=w268:i32)
              }
            }
            "ERRORES_T" <- w248
            n100 = call "Time Delay3"("error in (no error)"=w247, "Delay Time (s)"=2.0) -> ("error out"=w261:errorcluster)  [unwired: 9 in]
            n101 = local write "P116x2"(w245) -> ()
            n102 = global write "REACTOR_GLOBALES.vi" "P116x2"(w245) -> ()
            n103 = call <vilib>:"Simple Error Handler.vi"("error source (\" \")"=" \"cReadEurotherms\" " ("error source (\" \")"), "error in (no error)"=w261) -> ("error out"=w223:errorcluster)  [unwired: 3 in, 4 out]
          }
          frame "cLEER ALICATS" {
            # "LECTURA DE CONTROLADORES ALICAT EN RAMPA DE TEMPERATURA"
            # "LEER ALICATES"
            n104 = call "Display_Module.vi"("Command"=Display_Command_Control."Generate Event", "error in (no error)"=w315, "Data"="LEYENDO FLUJOS GASES ...", "Data Type"=Data_Type."Upd Status") -> ("error out"=w305:errorcluster)  [unwired: 7 in]
            n105 = call "__Alicat SD_ReadFlows.vi"("Nodos"=4, "error in"=w305, "COMMS"=w306) -> ("error out"=w304:errorcluster, "ParsedReadingArray"=w284:T3[], "aDispositivos 2"=w288:T4)  [unwired: 6 in]
            n106 = local write "ParsedReadingArray"(w284) -> ()
            n107 = Index Array(array=w288, index (col)=6 ("disabled index (col)")) -> (element=w300:string[])  [unwired: 1 in]
            n108 = Fract/Exp String To Number(string=w300) -> (number=w298:dbl[])  [unwired: 3 in, 1 out]
            n109 = Index Array(array=w298) -> (element #1=w296:dbl, element #2=w294:dbl, element #3=w293:dbl, element #4=w292:dbl)  [unwired: 4 in]
            n110 = Bundle By Name(cluster=w287, "a FSET1"=w296, "a FSET2"=w294, "a FSET3"=w293, "a FSET4"=w292) -> (w286:T6)
            n111 = Index Array(array=w288, index (col)=7 ("disabled index (col)")) -> (element=w299:string[])  [unwired: 1 in]
            n112 = Fract/Exp String To Number(string=w299) -> (number=w297:dbl[])  [unwired: 3 in, 1 out]
            n113 = Index Array(array=w297) -> (element #1=w295:dbl, element #2=w291:dbl, element #3=w290:dbl, element #4=w289:dbl)  [unwired: 5 in, 1 out]
            n114 = Bundle By Name(cluster=w286, "a FLUJO1"=w295, "a FLUJO2"=w291, "a FLUJO3"=w290, "a FLUJO4"=w289) -> (w285:T6)
            n115 = call "Time Delay21"("error in (no error)"=w304, "Delay Time (s)"=1.0) -> ("error out"=w307:errorcluster)  [unwired: 9 in]
            n116 = call <vilib>:"Simple Error Handler.vi"("error source (\" \")"=" \"cReadAlicats\" " ("error source (\" \")"), "error in (no error)"=w307) -> ("error out"=w312:errorcluster)  [unwired: 3 in, 4 out]
          }
          frame "cGUARDAR DATOS" {
            # "GUARDAR DATOS EN RAMPA DE TEMPERATURA"
            n117 = global read "REACTOR_GLOBALES.vi" "Comments"() -> (w319:string)
            n118 = call "File_Module.vi"("Command"=File_Module_Control."Save Data", "error in (no error)"=w331, "DATOS"=w324, "Comments"=w319) -> ("error out"=w325:errorcluster)  [unwired: 6 in, 1 out]
            n119 = call "Display_Module.vi"("Command"=Display_Command_Control."Generate Event", "error in (no error)"=w325, "Data"=w324, "Data Type"=Data_Type."Update FP") -> ("error out"=w321:errorcluster)  [unwired: 7 in]
            n120 = call <vilib>:"Simple Error Handler.vi"("error source (\" \")"=" \"cSaveDatos\" " ("error source (\" \")"), "error in (no error)"=w321) -> ("error out"=w320:errorcluster)  [unwired: 3 in, 4 out]
          }
          frame "cWAIT NEXT" {
            # "SIGUIENTE MUESTRA EN RAMPA DE TEMPERATURA"
            # "Espera x segundos"
            n121 = global read "REACTOR_GLOBALES.vi" "Muestreo(s)"() -> (w332:dbl)
            n122 = local write "Muestreo(s)"(w332) -> ()
            n123 = call "P2018 Elapsed_Sampling_Seconds_Module.vi"("Command"=Timing_Module_Control."Check Time", "error in (no error)"=w352, "Time In"=w332) -> ("error out"=w351:errorcluster, "Elapsed Out"=w348:dbl, "Time Elapsed"=w349:bool)  [unwired: 6 in]
            n124 = Subtract(x=w332, y=w348) -> (x-y=w341:dbl)
            n125 = Divide(x=w341, y=1.0) -> (x/y=w340:dbl)
            n126 = Number To Fractional String(number=w340, precision (6)=i16 1) -> (F-format string=w344:string)  [unwired: 2 in]
            n127 = local read "Timestring"() -> (w337:string)
            n128 = Concatenate Strings(w337, "; Siguiente muestra (s) ", w344) -> (w345:string)
            n129 = call "Display_Module.vi"("Command"=Display_Command_Control."Generate Event", "error in (no error)"=w351, "Data"=w345, "Data Type"=Data_Type."Upd Status") -> ("error out"=w350:errorcluster)  [unwired: 7 in]
            n130 = case shown="False" w349 {
              tunnel: [REACTOR_MODO_AUTOM."cWAIT NEXT" ("Command") REACTOR_MODO_AUTOM."cTEMPERATURA ESTABLE?" ("Command")] -> w355
              tunnel: w350 -> [w360 w363]
              tunnel: [w360 w362] -> w339
              frame False {
              }
              frame True {
                n131 = call "P2018 Elapsed_Sampling_Seconds_Module.vi"("Command"=Timing_Module_Control."Initialize Time", "error in (no error)"=w363) -> ("error out"=w362:errorcluster)  [unwired: 7 in, 2 out]
              }
            }
            n132 = call "Time Delay"("error in (no error)"=w339, "Delay Time (s)"=0.05) -> ("error out"=w334:errorcluster)  [unwired: 9 in]
            n133 = call <vilib>:"Simple Error Handler.vi"("error source (\" \")"=" \"cWait next\" " ("error source (\" \")"), "error in (no error)"=w334) -> ("error out"=w333:errorcluster)  [unwired: 3 in, 4 out]
          }
          frame "cTEMPERATURA ESTABLE?" {
            # "COMPROBAR SI LA TEMPERATURA ES ESTABLE"
            # "Tiempo para estabilizar: Delat_t (s). Ambas temperaturas estarán \ndentro de un margen de Delta_T (C) durante este tiempo\npara considerar que la temperatura es estable."
            # "Maximo tiempo para estabilizar: Max_t (s). \nTranscurrido este tiempo, se considerara estable, \npara no paralizar el programa"
            n134 = global read "REACTOR_GLOBALES.vi" "Delta_T (C)"() -> (w389:dbl)
            n135 = Unbundle By Name(w373) -> ("SET_TH"=w397:dbl, "TEMP_TH"=w396:dbl, "TEMP_TH"=w395:dbl, "TEMP_TC"=w394:dbl)
            n136 = Subtract(x=w397, y=w396) -> (x-y=w393:dbl)
            n137 = Subtract(x=w395, y=w394) -> (x-y=w392:dbl)
            n138 = Absolute Value(x=w393) -> (abs(x)=w391:dbl)
            n139 = Absolute Value(x=w392) -> (abs(x)=w390:dbl)
            n140 = Less?(x=w391, y=w389) -> (x < y?=w387:bool)
            n141 = Less?(x=w390, y=w389) -> (x < y?=w388:bool)
            n142 = And(x=w387, y=w388) -> (x .and. y?=w375:bool)
            n143 = case shown="True" w375 {
              tunnel: w367 -> [w403 w408]
              tunnel: [w402 w407] -> w378
              tunnel: [FALSE ("TStable?") w406] -> w374
              frame False {
                n144 = call "Elapsed_StableT_Minutes_Module.vi"("Command"=Timing_Module_Control."Initialize Time", "error in (no error)"=w403) -> ("error out"=w402:errorcluster)  [unwired: 7 in, 2 out]
              }
              frame True {
                n145 = global read "REACTOR_GLOBALES.vi" "Delta_t (s)"() -> (w405:dbl)
                n146 = call "Elapsed_StableT_Minutes_Module.vi"("Command"=Timing_Module_Control."Check Time", "error in (no error)"=w408, "Time In"=w405) -> ("error out"=w407:errorcluster, "Time Elapsed"=w406:bool)  [unwired: 6 in, 1 out]
              }
            }
            n147 = global read "REACTOR_GLOBALES.vi" "Max_t (s)"() -> (w379:dbl)
            n148 = Select(t=", SI", s=w375, f=", NO") -> (s? t:f=w381:string)
            n149 = call "Elapsed_Step_Minutes_Module.vi"("Command"=Timing_Module_Control."Check Time", "error in (no error)"=w378, "Time In"=w379) -> ("error out"=w368:errorcluster, "Elapsed Out"=w370:dbl, "Time Elapsed"=w377:bool)  [unwired: 6 in]
            n150 = Or(x=w374, y=w377) -> (x .or. y?=w376:bool)
            n151 = Number To Fractional String(number=w370, precision (6)=i16 1) -> (F-format string=w384:string)  [unwired: 2 in]
            n152 = Concatenate Strings("Estabilizando, t(s)   ", w384, w381) -> (w369:string)
            n153 = local write "Timestring"(w369) -> ()
            n154 = Select(t=REACTOR_MODO_AUTOM."TEST COMANDO" ("Command"), s=w376, f=REACTOR_MODO_AUTOM."cLEER TIEMPO" ("Command")) -> (s? t:f=w398:T9)
            n155 = call <vilib>:"Simple Error Handler.vi"("error source (\" \")"=" \"cEstableTemp?\" " ("error source (\" \")"), "error in (no error)"=w368) -> ("error out"=w371:errorcluster)  [unwired: 3 in, 4 out]
          }
          frame "CAMBIO TIEMPOS" {
            w416 = Timing_Module_Control."Initialize Time" ("Command")
            # "EXTRAE TIEMPO DE MEDIDA A TEMPERATURA CONSTANTE"
            # "Temperatura plato (T cte) en segundos"
            # "MANTENER temperatura constante durante 5.0min"
            # "Temperatura plato (T cte) en minutos"
            n156 = Index Array(array=w427, index=w426) -> (element=w428:string)
            n157 = Scan From String(format string="MANTENER temperatura constante durante %fmin", input string=w428) -> (output 1=w411:dbl)  [unwired: 3 in, 3 out]
            n158 = Multiply(x=w411, y=60.0) -> (x*y=w410:dbl)
            "tPlato(s)" <- w410
            n159 = global write "REACTOR_GLOBALES.vi" "tPlato(s)"(w410) -> ()
            n160 = call "P2018 Elapsed_Sampling_Seconds_Module.vi"("Command"=w416, "error in (no error)"=w422) -> ("error out"=w421:errorcluster)  [unwired: 7 in, 2 out]
            n161 = call "Elapsed_Step_Minutes_Module.vi"("Command"=w416, "error in (no error)"=w421) -> ("error out"=w417:errorcluster)  [unwired: 7 in, 2 out]
            n162 = call "Elapsed_StableT_Minutes_Module.vi"("Command"=w416, "error in (no error)"=w417) -> ("error out"=w413:errorcluster)  [unwired: 7 in, 2 out]
            n163 = call "Time Delay14"("error in (no error)"=w413, "Delay Time (s)"=0.05) -> ("error out"=w412:errorcluster)  [unwired: 9 in]
            n164 = call <vilib>:"Simple Error Handler.vi"("error source (\" \")"=" \"cambioTiempos\" " ("error source (\" \")"), "error in (no error)"=w412) -> ("error out"=w418:errorcluster)  [unwired: 3 in, 4 out]
          }
          frame "tLEER TIEMPO" {
            # "LEER TIEMPO ACTUAL CON TEMPERATURA CONSTANTE"
            # "Actualiza el tiempo para almacenarlo en fichero de datos"
            n165 = call "P2018 Elapsed_Total_Minutes_Module.vi"("Command"=Timing_Module_Control."Check Time", "error in (no error)"=w439) -> ("error out"=w431:errorcluster, "Elapsed Out"=w434:dbl)  [unwired: 7 in, 1 out]
            n166 = Bundle By Name(cluster=w443, "TIEMPO"=w434) -> (w440:T6)
            n167 = call "Time Delay16"("error in (no error)"=w431, "Delay Time (s)"=0.05) -> ("error out"=w430:errorcluster)  [unwired: 9 in]
            n168 = call <vilib>:"Simple Error Handler.vi"("error source (\" \")"="\"tReadTiempo\"" ("error source (\" \")"), "error in (no error)"=w430) -> ("error out"=w435:errorcluster)  [unwired: 3 in, 4 out]
          }
          frame "tLEER TEMPERATURAS" {
            w455 = T15 [enum."Add 1", enum."Add 2"] items=["Add 1", "Add 2", "Add 10", "Add 11", "Add 12", "Add 13"]
            # "NO CIERRA PUERTO"
            # "NO ABRE PUERTO"
            # "LECTURA DE CONTROLADORES EUROTHERM CON TEMPERATURA CONSTANTE"
            n169 = Unbundle By Name(w446) -> ("euro"=w479:bool, "Eurotherm"=w481:refnum<visa-resource-name>)
            n170 = call "Display_Module.vi"("Command"=Display_Command_Control."Generate Event", "error in (no error)"=w450, "Data"="LEYENDO TEMPERATURAS ...", "Data Type"=Data_Type."Upd Status") -> ("error out"=w468:errorcluster)  [unwired: 7 in]
            n171 = call "Eurotherm_New_Module.vi"("Eurotherm (T:Enable)"=FALSE, "Command"=Eurotherm_New_Module."Initialize", "error in (no error)"=w468, "VISA resource name"=w481) -> ("error out"=w478:errorcluster)  [unwired: 6 in, 1 out]
            n172 = for {
              tunnel: w455 -> [_] mode=indexing
              tunnel: [w504] -> w465 mode=indexing
              tunnel: [w503] -> w464 mode=indexing
              shift-right: [w501] -> w480
              shift-left: w478 -> [w497]
              tunnel: w479 -> [w493]
              tunnel: [w502] -> w477 mode=indexing
              tunnel: [w493] -> _
              tunnel: w481 -> [w492]
              tunnel: [w492] -> w482
              w494 = u16 1 items=["0"=1, "1"=10, "2"=100] ("Decimales")
              # "SELECT: targetSP o workingSP"
              n173 = call "Eurotherm_New_Module.vi"("Decimales"=w494, "Eurotherm (T:Enable)"=w493, "Command"=Eurotherm_New_Module."Read SP+PV", "error in (no error)"=w497, "VISA resource name"=w492) -> ("error out"=w498:errorcluster, "Eurotherm"=w495:T16)  [unwired: 5 in]
              n174 = call "coerceData.vi"("Eurotherm"=w495) -> ("Eurotherm 2"=w499:T16)  [unwired: 10 in]
              n175 = Unbundle By Name(w499) -> ("targetSP"=w504:dbl, "processVal"=w503:dbl, "workingOut"=w502:dbl)
              n176 = call "Time Delay13"("error in (no error)"=w498, "Delay Time (s)"=0.125) -> ("error out"=w501:errorcluster)  [unwired: 9 in]
            }
            n177 = Array To Cluster(array=w465) -> (cluster=w474:cluster{"[0]":dbl, "[1]":dbl})
            n178 = Array To Cluster(array=w464) -> (cluster=w473:cluster{"[0]":dbl, "[1]":dbl})
            n179 = Array To Cluster(array=w477) -> (cluster=w472:cluster{"[0]":dbl, "[1]":dbl})
            n180 = Index Array(array=w465) -> (element #1=w463:dbl, element #2=w462:dbl)  [unwired: 2 in]
            n181 = Index Array(array=w464) -> (element #1=w461:dbl, element #2=w460:dbl)  [unwired: 2 in]
            n182 = call "Eurotherm_New_Module.vi"("Eurotherm (T:Enable)"=FALSE, "Command"=Eurotherm_New_Module."Shutdown", "error in (no error)"=w480, "VISA resource name"=w482) -> ("error out"=w469:errorcluster)  [unwired: 6 in, 1 out]
            n183 = Bundle By Name(cluster=w449, "SET_TH"=w463, "SET_TC"=w462, "TEMP_TH"=w461, "TEMP_TC"=w460) -> (w448:T6)
            n184 = Unbundle By Name(w469) -> ("status"=w476:bool)
            n185 = local read "P116x2"() -> (w466:T1)
            n186 = Bundle By Name(cluster=w466, "TargetSP"=w474, "Temperatura"=w473, "Potencia"=w472, "Error"=w476) -> (w475:T1)
            n187 = local read "ERRORES_T 2"() -> (w471:i32)
            n188 = case shown="True" w476 {
              tunnel: w475 -> [w488 _]
              tunnel: [w488 w489] -> w467
              tunnel: w466 -> [_ w489]
              tunnel: w471 -> [w487 w491]
              tunnel: [w487 w490] -> w470
              frame False {
              }
              frame True {
                n189 = Increment(x=w491) -> (x+1=w490:i32)
              }
            }
            "ERRORES_T 2" <- w470
            n190 = call "Time Delay12"("error in (no error)"=w469, "Delay Time (s)"=2.0) -> ("error out"=w483:errorcluster)  [unwired: 9 in]
            n191 = local write "P116x2"(w467) -> ()
            n192 = global write "REACTOR_GLOBALES.vi" "P116x2"(w467) -> ()
            n193 = call <vilib>:"Simple Error Handler.vi"("error source (\" \")"=" \"tReadEurotherms\" " ("error source (\" \")"), "error in (no error)"=w483) -> ("error out"=w445:errorcluster)  [unwired: 3 in, 4 out]
          }
          frame "tLEER ALICATS" {
            # "LECTURA DE CONTROLADORES ALICAT CON TEMPERATURA CONSTANTE"
            # "SUSTITUIR POR LEER ALICATES"
            n194 = call "Display_Module.vi"("Command"=Display_Command_Control."Generate Event", "error in (no error)"=w537, "Data"="LEYENDO FLUJOS GASES...", "Data Type"=Data_Type."Upd Status") -> ("error out"=w527:errorcluster)  [unwired: 7 in]
            n195 = call "__Alicat SD_ReadFlows.vi"("Nodos"=4, "error in"=w527, "COMMS"=w528) -> ("error out"=w526:errorcluster, "ParsedReadingArray"=w506:T3[], "aDispositivos 2"=w510:T4)  [unwired: 6 in]
            n196 = local write "ParsedReadingArray"(w506) -> ()
            n197 = Index Array(array=w510, index (col)=6 ("disabled index (col)")) -> (element=w522:string[])  [unwired: 1 in]
            n198 = Fract/Exp String To Number(string=w522) -> (number=w520:dbl[])  [unwired: 3 in, 1 out]
            n199 = Index Array(array=w520) -> (element #1=w518:dbl, element #2=w516:dbl, element #3=w515:dbl, element #4=w514:dbl)  [unwired: 4 in]
            n200 = Bundle By Name(cluster=w509, "a FSET1"=w518, "a FSET2"=w516, "a FSET3"=w515, "a FSET4"=w514) -> (w508:T6)
            n201 = Index Array(array=w510, index (col)=7 ("disabled index (col)")) -> (element=w521:string[])  [unwired: 1 in]
            n202 = Fract/Exp String To Number(string=w521) -> (number=w519:dbl[])  [unwired: 3 in, 1 out]
            n203 = Index Array(array=w519) -> (element #1=w517:dbl, element #2=w513:dbl, element #3=w512:dbl, element #4=w511:dbl)  [unwired: 5 in, 1 out]
            n204 = Bundle By Name(cluster=w508, "a FLUJO1"=w517, "a FLUJO2"=w513, "a FLUJO3"=w512, "a FLUJO4"=w511) -> (w507:T6)
            n205 = call "Time Delay9"("error in (no error)"=w526, "Delay Time (s)"=1.0) -> ("error out"=w529:errorcluster)  [unwired: 9 in]
            n206 = call <vilib>:"Simple Error Handler.vi"("error source (\" \")"=" \"tReadAlicats\" " ("error source (\" \")"), "error in (no error)"=w529) -> ("error out"=w534:errorcluster)  [unwired: 3 in, 4 out]
          }
          frame "tGUARDAR DATOS" {
            # "GUARDAR DATOS CON TEMPERATURA CONSTANTE"
            n207 = global read "REACTOR_GLOBALES.vi" "Comments"() -> (w544:string)
            n208 = call "File_Module.vi"("Command"=File_Module_Control."Save Data", "error in (no error)"=w555, "DATOS"=w548, "Comments"=w544) -> ("error out"=w549:errorcluster)  [unwired: 6 in, 1 out]
            n209 = call "Display_Module.vi"("Command"=Display_Command_Control."Generate Event", "error in (no error)"=w549, "Data"=w548, "Data Type"=Data_Type."Update FP") -> ("error out"=w541:errorcluster)  [unwired: 7 in]
            n210 = call "Time Delay10"("error in (no error)"=w541, "Delay Time (s)"=0.05) -> ("error out"=w540:errorcluster)  [unwired: 9 in]
            n211 = call <vilib>:"Simple Error Handler.vi"("error source (\" \")"=" \"tSaveDatos\" " ("error source (\" \")"), "error in (no error)"=w540) -> ("error out"=w545:errorcluster)  [unwired: 3 in, 4 out]
          }
          frame "tWAIT NEXT" {
            # "AGOTADO TIEMPO CON TEMPERATURA CONSTANTE"
            # "Espera x segundos"
            n212 = global read "REACTOR_GLOBALES.vi" "Muestreo(s)"() -> (w556:dbl)
            n213 = local write "Muestreo(s)"(w556) -> ()
            n214 = call "P2018 Elapsed_Sampling_Seconds_Module.vi"("Command"=Timing_Module_Control."Check Time", "error in (no error)"=w577, "Time In"=w556) -> ("error out"=w576:errorcluster, "Elapsed Out"=w575:dbl, "Time Elapsed"=w560:bool)  [unwired: 6 in]
            n215 = Subtract(x=w556, y=w575) -> (x-y=w564:dbl)
            n216 = Number To Fractional String(number=w564, precision (6)=i16 1) -> (F-format string=w571:string)  [unwired: 2 in]
            n217 = local read "Timestring"() -> (w563:string)
            n218 = Concatenate Strings(w563, ", Siguiente muestra (s) ", w571) -> (w572:string)
            n219 = call "Display_Module.vi"("Command"=Display_Command_Control."Generate Event", "error in (no error)"=w576, "Data"=w572, "Data Type"=Data_Type."Upd Status") -> ("error out"=w559:errorcluster)  [unwired: 7 in]
            n220 = case shown="True" w560 {
              tunnel: [REACTOR_MODO_AUTOM."tWAIT NEXT" ("Command") REACTOR_MODO_AUTOM."tAGOTADO TIEMPO?" ("Command")] -> w557
              tunnel: w559 -> [w584 w586]
              tunnel: [w584 w585] -> w558
              frame False {
              }
              frame True {
                n221 = call "P2018 Elapsed_Sampling_Seconds_Module.vi"("Command"=Timing_Module_Control."Initialize Time", "error in (no error)"=w586) -> ("error out"=w585:errorcluster)  [unwired: 7 in, 2 out]
              }
            }
            n222 = Select(t=REACTOR_MODO_AUTOM."TEST COMANDO" ("Command"), s=w560, f=REACTOR_MODO_AUTOM."tLEER TIEMPO" ("Command")) -> ()  [unwired: 1 out]
            n223 = call "Time Delay8"("error in (no error)"=w558, "Delay Time (s)"=0.05) -> ("error out"=w566:errorcluster)  [unwired: 9 in]
            n224 = call <vilib>:"Simple Error Handler.vi"("error source (\" \")"=" \"tWait next\" " ("error source (\" \")"), "error in (no error)"=w566) -> ("error out"=w565:errorcluster)  [unwired: 3 in, 4 out]
          }
          frame "tAGOTADO TIEMPO?" {
            # "SIGUIENTE MUESTRA CON TEMPERATURA CONSTANTE"
            # "Si pulsamos boton SALTAR, finalizamos este paso del programa"
            n225 = local read "tPlato(s)"() -> (w594:dbl)
            n226 = global read "REACTOR_GLOBALES.vi" "PAUSA"() -> (w602:bool)
            n227 = case shown="True" w602 {
              tunnel: w594 -> [w617 _]
              tunnel: [w617 1000000.0] -> w601
              frame False {
              }
              frame True {
              }
            }
            n228 = call "Elapsed_Step_Minutes_Module.vi"("Command"=Timing_Module_Control."Check Time", "error in (no error)"=w613, "Time In"=w601) -> ("error out"=w591:errorcluster, "Elapsed Out"=w611:dbl, "Time Elapsed"=w612:bool)  [unwired: 6 in]
            n229 = Subtract(x=w601, y=w611) -> (x-y=w605:dbl)
            n230 = Divide(x=w605, y=60.0) -> (x/y=w604:dbl)
            n231 = Number To Fractional String(number=w604, precision (6)=i16 1) -> (F-format string=w608:string)  [unwired: 2 in]
            n232 = Concatenate Strings("Tiempo de medida (min) ", w608) -> (w597:string)
            n233 = local write "Timestring"(w597) -> ()
            n234 = global read "REACTOR_GLOBALES.vi" "SALTAR"() -> (w603:bool)
            n235 = Or(x=w612, y=w603) -> (x .or. y?=w590:bool)
            n236 = Select(t=REACTOR_MODO_AUTOM."TEST COMANDO" ("Command"), s=w590, f=REACTOR_MODO_AUTOM."tLEER TIEMPO" ("Command")) -> (s? t:f=w589:T9)
            n237 = call "Time Delay11"("error in (no error)"=w591, "Delay Time (s)"=0.05) -> ("error out"=w595:errorcluster)  [unwired: 9 in]
            n238 = call <vilib>:"Simple Error Handler.vi"("error source (\" \")"=" \"tAgotadoTiempo?\" " ("error source (\" \")"), "error in (no error)"=w595) -> ("error out"=w598:errorcluster)  [unwired: 3 in, 4 out]
          }
          frame "FINALIZAR" {
            # "FINALIZAR AUTOMATICO"
            n239 = call "Display_Module.vi"("Command"=Display_Command_Control."Generate Event", "error in (no error)"=w630, "Data"="Fin de programa", "Data Type"=Data_Type."Upd Status") -> ("error out"=w625:errorcluster)  [unwired: 7 in]
            n240 = global write "REACTOR_GLOBALES.vi" "stop"(TRUE ("stop")) -> ()
            n241 = call "Display_Module.vi"("Command"=Display_Command_Control."Generate Event", "error in (no error)"=w625, "Data"=0, "Data Type"=Data_Type."En/Dis FP Ctls") -> ("error out"=w622:errorcluster)  [unwired: 7 in]
            n242 = call <vilib>:"Simple Error Handler.vi"("error source (\" \")"=" \"finalizar\" " ("error source (\" \")"), "error in (no error)"=w622) -> ("error out"=w621:errorcluster)  [unwired: 3 in, 4 out]
          }
        }
        "Datos" <- w34
        "TStable" <- w31
        n243 = call "REACTOR_STOP.vi"("error in (no error)"=w28, "Stop"=enum16{"Continue", "Stop", "Default"}."Default") -> ("error out"=w27:errorcluster, "Stop?"=w26:bool)  [unwired: 8 in]
        n244 = global write "REACTOR_GLOBALES.vi" "T ESTABLE?"(w31) -> ()
        n245 = Or(x=w26, y=w42) -> (x .or. y?=w43:bool)
        n246 = Wait (ms)(milliseconds to wait=u32 10) -> ()  [unwired: 1 out]
      }
    }
    frame Error {
    }
  }
  n247 = local read "Datos"() -> (w2:T6)
  n248 = call "Display_Module.vi"("Command"=Display_Command_Control."Generate Event", "error in (no error)"=w1, "Data"=w2, "Data Type"=Data_Type."Update FP") -> ("error out"=w3:errorcluster)  [unwired: 7 in]
  n249 = call "Display_Module.vi"("Command"=Display_Command_Control."Generate Event", "error in (no error)"=w3, "Data"="Fin de programa", "Data Type"=Data_Type."Upd Status") -> ("error out"=w17:errorcluster)  [unwired: 7 in]
  n250 = call "Display_Module.vi"("Command"=Display_Command_Control."Generate Event", "error in (no error)"=w17, "Data"=0, "Data Type"=Data_Type."En/Dis FP Ctls") -> ("error out"=w7:errorcluster)  [unwired: 7 in]
  n251 = call "REACTOR_STOP.vi"("error in (no error)"=w7, "Stop"=enum16{"Continue", "Stop", "Default"}."Continue") -> ("error out"=→"error out":errorcluster)  [unwired: 8 in, 1 out]
